vi "FPGA_test_QPD.vi"() -> ()   [LabVIEW 2015]
uses:
  <vilib>/Platform/TimedLoop/XDataNode/timing_clust.ctl
  <vilib>/Platform/TimedLoop/XDataNode/nitl_modes.ctl
  <vilib>/Platform/TimedLoop/XDataNode/wakeup.ctl
  <vilib>/rvi/FXPMathLib/basic elements/FxpIntAccumulator/subVIs/nifxpmath_IntAccumulator_SimConfig.ctl
  <vilib>/rvi/Emulation/niFpgaGetClockAttributes.vi
  <vilib>/rvi/Emulation/niFpgaSctlEmulationGetInTimedLoop.vi
  <vilib>/rvi/Emulation/niFpgaEmulationReportErrorSimple.vi
  <vilib>/rvi/eio/common/nirviEmuTemplateMethod_errors.vi
  <vilib>/rvi/Emulation/niFpgaProcessEmulError.vi
  <vilib>/rvi/Analysis/common/codeGenErrors/XNode/niFpgaXNodeCodeGenErrorHandle.vi
  <vilib>/rvi/Emulation/niFpgaCriticalErrorInLSC.vi
  <vilib>/rvi/FXPMathLib/basic elements/FxpIntAccumulator/simVIs/DllFxpIntAccumulator_sub.vi
  <vilib>/eio/EIONode/EIONode.xnode
  <vilib>/rvi/Analysis/measure/dc-rms/XNode/niFpgaDC-RMS.xnode
  <vilib>/Platform/TimedLoop/XDataNode/XDataNode.xnode
  <vilib>/rvi/FXPMathLib/basic elements/FxpIntAccumulator/XNode/nifxpmath_IntAccumulator.xnode
  <vilib>/rvi/FXPMathLib/FxpMul/XNode/nifxpmath_Multiplier.xnode
  <vilib>/Platform/TimedLoop/XDataNode/XDNodeRunTimeDep.lvlib
  <vilib>/rvi/FXPMathLib/sim/FxpSim.dll
panel:
  out "Waveform Chart":i16(graph)
  in  "Reset counter":bool
  out "QPD":T1
  in  "Count(uSec)":u32=100
  out "duration (ms)":u32
  in  "stop":bool
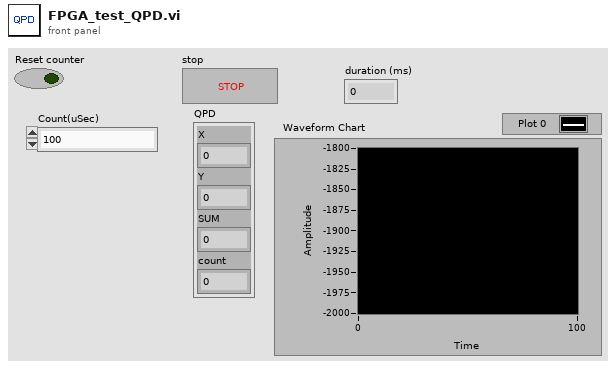
[diagram p1: front panel]
types:
  T1 = cluster{"X":sgl, "Y":sgl, "SUM":sgl, "count":u32}
  T2 = typedef "XDNodeRunTimeDep.lvlib/timing_clust.ctl" = cluster{"Expected End [f-1]":u64, "Actual End [f-1]":u64, "Finished Late? [f-1]":bool, "Expected End [i-1]":u64, "Actual End [i-1]":u64, "Finished Late? [i-1]":bool, "Expected Start [i]":u64, "Actual Start [i]":u64, "Expected Start [f]":u64, "Actual Start [f]":u64, "Source Name":string, "Structure Name":string, "Period":i64, "Deadline":i64, "Offset":i64, "Start":i64, "Priority":i32, "Timeout":i32, "Mode":T3, "Wakeup Reason":T4, "Error":errorcluster, "Source Type":string, "Secondary Source Type":string, "Global End Time":u64, "Global Start Time":u64, "Frame Duration":u64, "Iteration Duration":u64, "Assigned CPU":i32, "I/O Scan Engine Mode":u32}
  T3 = typedef "XDNodeRunTimeDep.lvlib/nitl_modes.ctl" = enum32{"No Change", "Process missed periods, maintain original phase", "Discard missed periods, maintain original phase", "Process missed periods, ignore original phase", "Discard missed periods, ignore original phase"}
  T4 = typedef "XDNodeRunTimeDep.lvlib/wakeup.ctl" = enum32{"Normal", "Aborted", "Asynchronous wakeup", "Timing source error", "Timed loop error", "Timeout"}
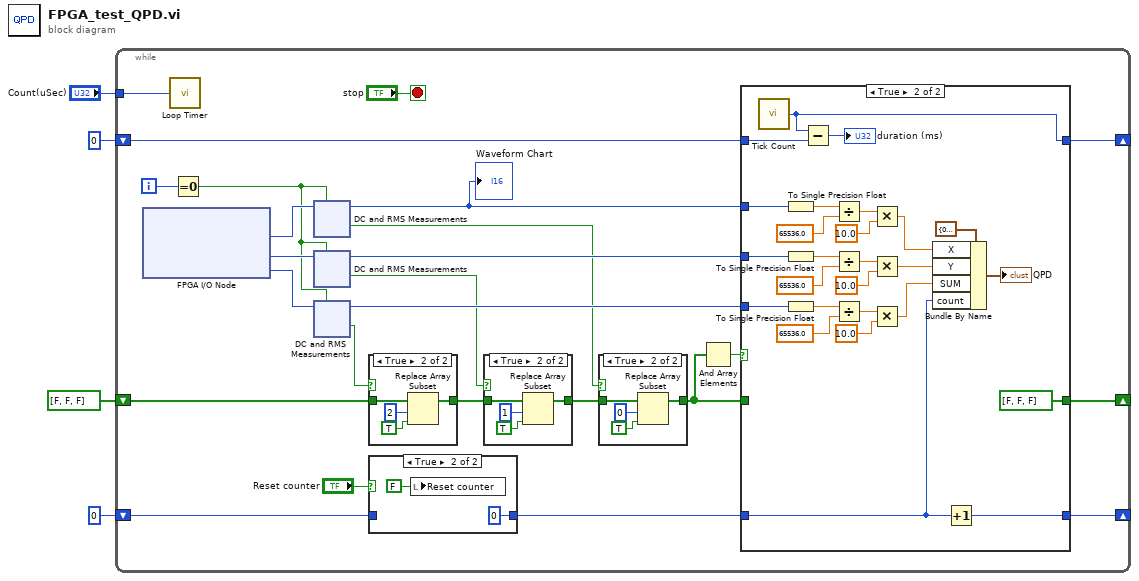
[diagram p0: block diagram]
diagram:
  n1 = while {
    shift-right: [w13] -> _
    shift-left: bool[] [FALSE, FALSE, FALSE] ("initialized array") -> [w21]
    shift-right: [w11] -> _
    shift-left: u32 0 -> [w12]
    tunnel: "Count(uSec)" -> [w10]
    shift-right: [w9] -> _
    shift-left: u32 0 -> [w7]
    i -> [w27]
    stop <- "stop" stop-if-true
    n2 = xnode "FPGA I/O Node"() -> ("Connector0/AI0"=w29:i16, "Connector0/AI1"=w26:i16, "Connector0/AI2"=w25:i16)  [unwired: 3 in, 3 out]
    n3 = call "Loop Timer"("Count(uSec)"=w10) -> ()  [unwired: 1 out]
    n4 = Equal To 0?(x=w27) -> (x = 0?=w22:bool)
    n5 = xnode "DC and RMS Measurements"("input data"=w29, "reset"=w22) -> ("DC"=w5:i16, "output valid"=w16:bool)
    "Waveform Chart" <- w5
    n6 = xnode "DC and RMS Measurements"("input data"=w26, "reset"=w22) -> ("DC"=w24:i16, "output valid"=w17:bool)
    n7 = xnode "DC and RMS Measurements"("input data"=w25, "reset"=w22) -> ("DC"=w23:i16, "output valid"=w18:bool)
    n8 = case shown="True" w18 {
      tunnel: w21 -> [w38 w41]
      tunnel: [w38 w39] -> w20
      frame False {
      }
      frame True {
        n9 = Replace Array Subset(array=w41, new element=TRUE, index=2) -> (w39:bool[])
      }
    }
    n10 = case shown="True" "Reset counter" {
      tunnel: w7 -> [w30 _]
      tunnel: [w30 u32 0] -> w6
      frame False {
      }
      frame True {
        n11 = local write "Reset counter"(FALSE ("Reset counter")) -> ()
      }
    }
    n12 = case shown="True" w17 {
      tunnel: w20 -> [w43 w46]
      tunnel: [w43 w44] -> w19
      frame False {
      }
      frame True {
        n13 = Replace Array Subset(array=w46, new element=TRUE, index=1) -> (w44:bool[])
      }
    }
    n14 = case shown="True" w16 {
      tunnel: [w33 w35] -> w14
      tunnel: w19 -> [w33 w34]
      frame False {
      }
      frame True {
        n15 = Replace Array Subset(array=w34, new element=TRUE, index=0) -> (w35:bool[])
      }
    }
    n16 = And Array Elements(Boolean array=w14) -> (logical AND=w15:bool)
    n17 = case shown="True" w15 {
      tunnel: w5 -> [_ w76]
      tunnel: w24 -> [_ w67]
      tunnel: w23 -> [_ w62]
      tunnel: w14 -> [w50 _]
      tunnel: [w50 bool[] [FALSE, FALSE, FALSE] ("initialized array")] -> w13
      tunnel: w12 -> [w49 w57]
      tunnel: [w49 w55] -> w11
      tunnel: w6 -> [w48 w52]
      tunnel: [w48 w51] -> w9
      frame False {
      }
      frame True {
        n18 = call "Tick Count"() -> ("Tick Count(mSec)"=w55:u32)
        n19 = To Single Precision Float(number=w76) -> (single precision float=w75:sgl)
        n20 = To Single Precision Float(number=w67) -> (single precision float=w68:sgl)
        n21 = To Single Precision Float(number=w62) -> (single precision float=w66:sgl)
        n22 = Subtract(x=w55, y=w57) -> (x-y=→"duration (ms)":u32)
        n23 = Divide(x=w75, y=sgl 65536.0) -> (x/y=w73:sgl)
        n24 = Divide(x=w68, y=sgl 65536.0) -> (x/y=w70:sgl)
        n25 = Divide(x=w66, y=sgl 65536.0) -> (x/y=w64:sgl)
        n26 = Multiply(x=w73, y=sgl 10.0) -> (x*y=w61:sgl)
        n27 = Multiply(x=w70, y=sgl 10.0) -> (x*y=w60:sgl)
        n28 = Multiply(x=w64, y=sgl 10.0) -> (x*y=w59:sgl)
        n29 = Bundle By Name(cluster=T1 {"X"=0.0, "Y"=0.0, "SUM"=0.0, "count"=0} ("output cluster"), "X"=w61, "Y"=w60, "SUM"=w59, "count"=w52) -> (→"QPD":T1)
        n30 = Increment(x=w52) -> (x+1=w51:u32)
      }
    }
  }
